vi "Create Item.vi"(8 "error in (no error)":errorcluster caption="错误输入（无错误）", 9 "ImageIndex":i32, 10 "Width":i32, 11 "text":string) -> (0 "error out":errorcluster caption="错误输出", 2 "ItemRef":refnum<k24>, 3 "ToolStripLabel 输出":refnum<class "ToolStripLabel.lvclass"> caption="DNL_LabVIEW Object out")   [LabVIEW 2013, in "ToolStripLabel.lvclass"]
uses:
  ToolStripLabel.lvclass
  System.Windows.Forms
  System.Drawing
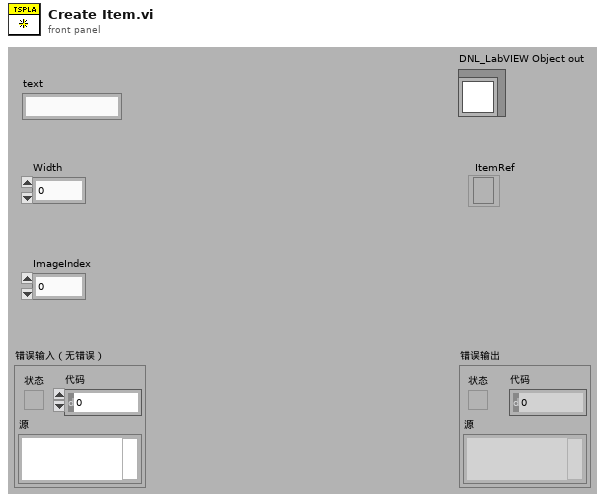
[diagram p1: front panel]
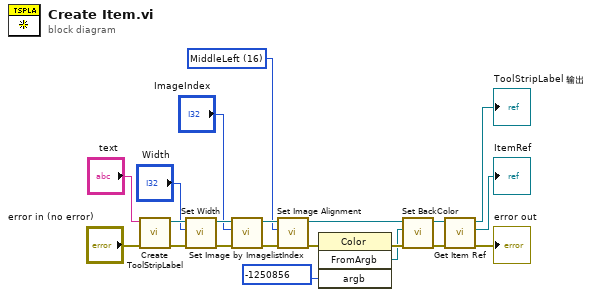
[diagram p0: block diagram]
diagram:
  w3 = 16 items=["TopLeft"=1, "TopCenter"=2, "TopRight"=4, "MiddleLeft"=16, "MiddleCenter"=32, "MiddleRight"=64, "BottomLeft"=256, "BottomCenter"=512, "BottomRight"=1024] ("ImageAlign")
  n1 = call "Create ToolStripLabel.vi"("error in (no error)"="error in (no error)", "text"="text") -> ("error out"=w20:errorcluster, "ToolStripLabel 输出"=w16:refnum<class "ToolStripLabel.lvclass">)  [unwired: 8 in]
  n2 = call "Set Width.vi"("error in (no error)"=w20, "Width"="Width", "ToolStripLabel 输入"=w16) -> ("error out"=w19:errorcluster, "ToolStripLabel 输出"=w14:refnum<class "ToolStripLabel.lvclass">)  [unwired: 7 in]
  n3 = call "Set Image by ImagelistIndex.vi"("error in (no error)"=w19, "ImageIndex"="ImageIndex", "ToolStripLabel 输入"=w14) -> ("error out"=w4:errorcluster, "ToolStripLabel 输出"=w5:refnum<class "ToolStripLabel.lvclass">)  [unwired: 7 in]
  n4 = call "Set Image Alignment.vi"("error in (no error)"=w4, "ImageAlign"=w3, "ToolStripLabel 输入"=w5) -> ("error out"=w2:errorcluster, "ToolStripLabel 输出"=w1:refnum<class "ToolStripLabel.lvclass">)  [unwired: 7 in]
  n5 = invoke class="Color" method="FromArgb"(error in=w2, "argb"=-1250856 ("ToArgb")) -> (error out=w8:errorcluster, "FromArgb"=w6:refnum<k24>)  [unwired: 2 in, 2 out]
  n6 = call "Set BackColor.vi"("error in (no error)"=w8, "BackColor"=w6, "ToolStripLabel 输入"=w1) -> ("error out"=w9:errorcluster, "ToolStripLabel 输出"=w10:refnum<class "ToolStripLabel.lvclass">)  [unwired: 7 in]
  n7 = call "Get Item Ref.vi"("error in (no error)"=w9, "ToolStripLabel 输入"=w10) -> ("error out"=→"error out":errorcluster, "ItemRef"=→"ItemRef":refnum<k24>, "ToolStripLabel 输出"=→"ToolStripLabel 输出":refnum<class "ToolStripLabel.lvclass">)  [unwired: 7 in]
